vi "Set Temp Control--Method.vi"(8 "Error In":errorcluster, 10 "Temp Control":bool, 11 "Watlow F4T in":refnum<class "Watlow F4T.lvclass">) -> (0 "Error Out":errorcluster, 3 "Watlow F4T out":refnum<class "Watlow F4T.lvclass">)   [LabVIEW 2024, in "Watlow F4T.lvclass"]
uses:
  Watlow F4T.lvclass
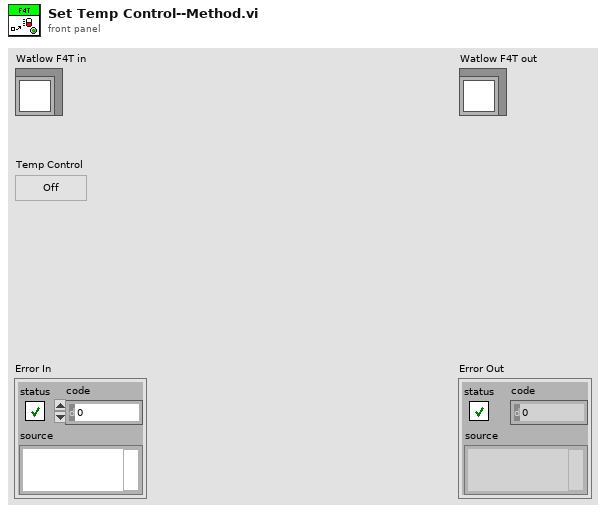
[diagram p1: front panel]
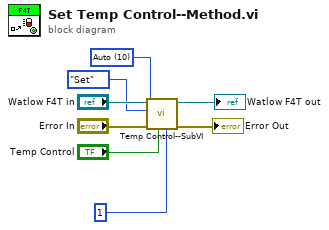
[diagram p0: block diagram]
diagram:
  w1 = u16 10 items=["Off"=62, "Auto"=10, "Manual"=54] ("Control Mode (Auto)")
  n1 = call "Temp Control--SubVI.vi"("Instance"=1, "Temp Control in"="Temp Control", "error in"="Error In", "Control Mode (Auto)"=w1, "Get/Set"=enum16{"Get", "Set"}."Set", "Watlow F4T in"="Watlow F4T in") -> ("error out"=→"Error Out":errorcluster, "Watlow F4T out"=→"Watlow F4T out":refnum<class "Watlow F4T.lvclass">)  [unwired: 3 in, 1 out]
